vi "AFT Destroy Adaptive Filter.vi"(8 "error in (no error)":errorcluster, 11 "adaptive filter in":refnum<k20>) -> (0 "error out":errorcluster)   [LabVIEW 2017, in "NI_AdaptiveFilter.lvlib"]
doc: "Destroys an adaptive filter. This VI releases all resources that the adaptive filter reserves."
uses:
  <vilib>/addons/Adaptive Filters/NI_AdaptiveFilter.lvlib
  <resource>/AdaptiveFilters.dll
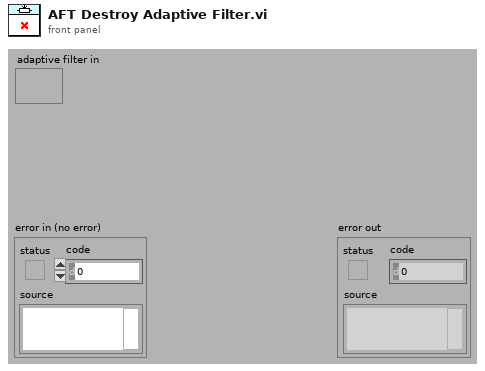
[diagram p1: front panel]
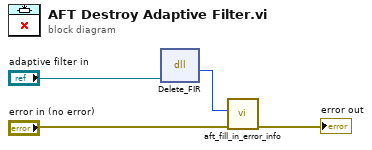
[diagram p0: block diagram]
diagram:
  n1 = dll-call lib="C:/Program Files/National Instruments/LabVIEW 2017/resource/AdaptiveFilters.dll" fn="Delete_FIR" ("Complex Data Initialization")("pSession"="adaptive filter in") -> ("err"=w1:i32)  [unwired: 4 in, 2 out]
  n2 = call <vilib>:"aft_fill_in_error_info.vi"("error in"="error in (no error)", "status code"=w1) -> ("error out"=→"error out":errorcluster)  [unwired: 2 in, 7 out]
